vi "Add Subaddress to Remote Terminal.vi"(4 "create timestamp channel":bool, 5 "remote terminal":T2, 6 "parameters":T5(array[cluster]), 7 "number of words":u16, 8 "error in":errorcluster, 9 "direction":T6, 10 "name":string, 11 "port":T1 format="%.0x") -> (0 "error out":errorcluster, 2 "subaddress":T1=18446744073709551615 format="%.0x", 3 "port out":T1 format="%.0x")   [LabVIEW 2020, in "AIM MIL-STD-1553 Scripting.lvlib"]
doc: "Adds a new <b>subaddress</b> with the specified <b>name</b> to a specified <b>remote terminal</b> in the <b>port</b>. Then performs the following in the Subaddress Section:\n1. If <b>remote terminal</b>::subaddress is 1-30, adds a Subaddress. If <b>remote terminal</b>::subaddress is 31, adds a Message Section (31 is reserved).\n2. Sets the <b>number of words</b> property for the Subaddress Section.\n3. Adds a Parameter Channel with the specified <b>direction</b> for each item in <b>parameters</b>.\n4. Creates a Timestamp channel if <b>create timestamp channel</b> is True."
uses:
  AIM MIL-STD-1553 Scripting.lvlib
  Shared/Direction.ctl
  Shared/Parameter Definition.ctl
  Shared/Terminal Endpoint.ctl
  Shared/Address.ctl
  <vilib>/NI VeriStand/Custom Device API/Custom Device Item Ref.ctl
  <vilib>/NI VeriStand/Custom Device API/Custom Device API.lvlib
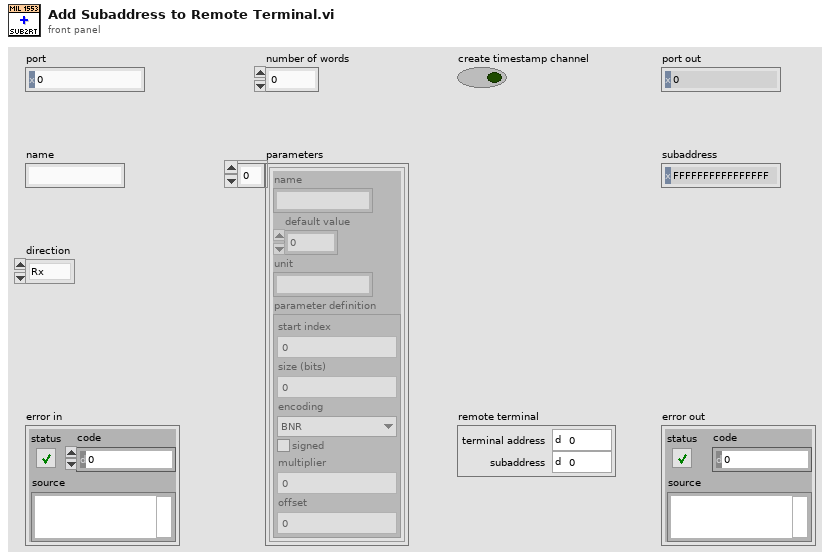
[diagram p1: front panel]
types:
  T1 = typedef "Custom Device API.lvlib/Custom Device Item Ref.ctl" = u64
  T2 = typedef "Terminal Endpoint.ctl" = cluster{"terminal address":T3, "subaddress":T3}
  T3 = typedef "Address.ctl" = u16
  T4 = typedef "Parameter Definition.ctl" = cluster{"start index":i32, "size (bits)":i32, "encoding":enum16{"BNR", "BCD", "Discrete"}, "signed":bool, "multiplier":dbl, "offset":dbl}
  T5 = cluster{"name":string, "default value":dbl, "unit":string, "parameter definition":T4}[]
  T6 = typedef "Direction.ctl" = enum16{"Rx", "Tx"}
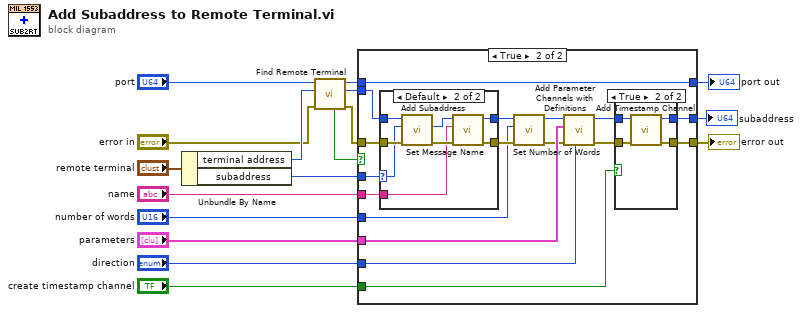
[diagram p0: block diagram]
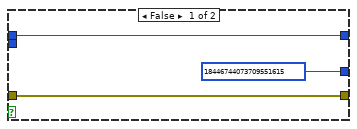
[diagram p2: hidden frame]
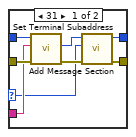
[diagram p3: hidden frame]
diagram:
  n1 = Unbundle By Name("remote terminal") -> ("terminal address"=w10:T3, "subaddress"=w12:T3)
  n2 = call "Find Remote Terminal.vi"("error in"="error in", "terminal address"=w10, "port"="port") -> ("error out"=w2:errorcluster, "remote terminal"=w3:T1, "port out"=w4:T1, "found?"=w5:bool)  [unwired: 5 in]
  n3 = case shown="True" w5 {
    tunnel: w4 -> [w20 w23]
    tunnel: w3 -> [_ w36]
    tunnel: w2 -> [w19 w37]
    tunnel: [w19 w26] -> w9
    tunnel: [w20 w23] -> w8
    tunnel: w12 -> [_ w35]
    tunnel: "number of words" -> [_ w28]
    tunnel: "parameters" -> [_ w34]
    tunnel: "name" -> [_ w29]
    tunnel: "direction" -> [_ w27]
    tunnel: "create timestamp channel" -> [_ w24]
    tunnel: [T1 18446744073709551615 ("message out") w21] -> w1
    frame False {
    }
    frame True {
      n4 = case shown="Default" w35 {
        selector: w35 -> [w38 w51]
        tunnel: w37 -> [w44 w53]
        tunnel: w36 -> [w45 w52]
        tunnel: [w41 w48] -> w33
        tunnel: [w39 w47] -> w32
        tunnel: w29 -> [w43 w46]
        frame 31 {
          n5 = call "Add Message Section.vi"("error in"=w44, "message section name"=w43, "bus controller"=w45) -> ("error out"=w40:errorcluster, "message section"=w42:T1)  [unwired: 6 in, 1 out]
          n6 = call "Set Terminal Subaddress.vi"("error in"=w40, "subaddress"=w38, "subaddress section"=w42) -> ("error out"=w39:errorcluster, "subaddress section out"=w41:T1)  [unwired: 7 in]
        }
        frame Default {
          n7 = call "Add Subaddress.vi"("error in"=w53, "subaddress"=w51, "remote terminal"=w52) -> ("error out"=w49:errorcluster, "subaddress section"=w50:T1)  [unwired: 6 in, 1 out]
          n8 = call "Set Message Name.vi"("error in"=w49, "name"=w46, "message or subaddress"=w50) -> ("error out"=w47:errorcluster, "message or subaddress out"=w48:T1)  [unwired: 7 in]
        }
      }
      n9 = call "Set Number of Words.vi"("error in"=w32, "number of words"=w28, "message or subaddress"=w33) -> ("error out"=w30:errorcluster, "message or subaddress out"=w31:T1)  [unwired: 7 in]
      n10 = call "Add Parameter Channels with Definitions.vi"("direction"=w27, "error in"=w30, "parameters"=w34, "message or subaddress"=w31) -> ("error out"=w25:errorcluster, "message or subaddress out"=w22:T1)  [unwired: 6 in]
      n11 = case shown="True" w24 {
        tunnel: w25 -> [w55 w59]
        tunnel: w22 -> [w54 w58]
        tunnel: [w55 w57] -> w26
        tunnel: [w54 w56] -> w21
        frame False {
        }
        frame True {
          n12 = call "Add Timestamp Channel.vi"("error in"=w59, "message section"=w58) -> ("error out"=w57:errorcluster, "message section out"=w56:T1)  [unwired: 7 in, 1 out]
        }
      }
    }
  }
  "error out" <- w9
  "port out" <- w8
  "subaddress" <- w1
